vi "Initialize.vi"(11 "Path to Secret Client JSON":path) -> (0 "error out":errorcluster, 3 "Google Drive Service Ref":refnum<k24>)   [LabVIEW 2018, in "GDrive.lvlib"]
doc: "This VI creates the authentication for the Google Drive. The first time that this VI executes, the user should see a prompt in a web browser that asks for access permission. After this first execution, this VI is required for flow because the Google Drive Service Reference contains the authorization required for the execution of other functions of this toolkit."
uses:
  GDrive.lvlib
  Y:/UCLA Google Drive/Xavier's Retina MBP/LabVIEW/GDrive/Dependencies/Google.Apis.Drive.v3.dll
  Dependencies/Google.Apis.Drive.v3.dll
  Y:/UCLA Google Drive/Xavier's Retina MBP/LabVIEW/GDrive/Dependencies/testAuth.dll
  Dependencies/testAuth.dll
panel:
  # "This VI authenticates a User's Google Drive account."
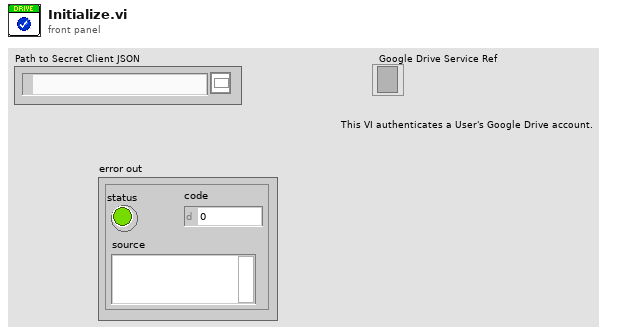
[diagram p1: front panel]
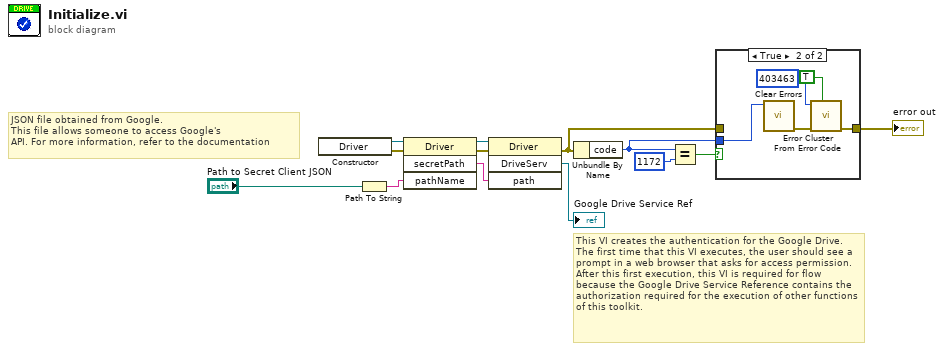
[diagram p0: block diagram]
diagram:
  # "JSON file obtained from Google.\nThis file allows someone to access Google's\nAPI. For more information, refer to the documentation"
  # "This VI creates the authentication for the Google Drive. The first time that this VI executes, the user should see a prompt in a web browser that asks for access permission. After this first execution, this VI is required for flow because the Google Drive Service Reference contains the authorization required for the execution of other functions of this toolkit."
  n1 = constructor class="Driver"() -> (reference out=w11:refnum<k24>, error out=w9:errorcluster)  [unwired: 3 in, 1 out]
  n2 = Path To String(path="Path to Secret Client JSON") -> (string=w7:string)
  n3 = invoke class="Driver" method="secretPath"(reference=w11, error in=w9, "pathName"=w7) -> (reference out=w12:refnum<k24>, error out=w8:errorcluster, "secretPath"=w13:string)  [unwired: 1 in, 1 out]
  n4 = invoke class="Driver" method="DriveServ"(reference=w12, error in=w8, "path"=w13) -> (error out=w2:errorcluster, "DriveServ"=→"Google Drive Service Ref":refnum<k24>)  [unwired: 1 in, 2 out]
  n5 = Unbundle By Name(w2) -> ("code"=w3:i32)
  n6 = Equal?(x=w3, y=1172) -> (x = y?=w5:bool)
  n7 = case shown="True" w5 {
    tunnel: w3 -> [_ w19]
    tunnel: w2 -> [w14 _]
    tunnel: [w14 w17] -> w1
    frame False {
    }
    frame True {
      n8 = call <vilib>:"Clear Errors.vi"("specific error code to clear (0: all)"=w19) -> ("error out"=w18:errorcluster)  [unwired: 5 in, 1 out]
      n9 = call <vilib>:"Error Cluster From Error Code.vi"("show call chain? (False)"=TRUE, "error in (no error)"=w18, "error code (0)"=403463) -> ("error out"=w17:errorcluster)  [unwired: 6 in]
    }
  }
  "error out" <- w1
